vi "RT Initialize Input Image (SubVI).vi"(8 "error in (no error)":errorcluster, 10 "Image Type":T2 items=["Grayscale (U8)", "Grayscale (I16)", "Grayscale (SGL)", "Complex (CSG)", "RGB (U32)", "HSL (U32)", "RGB (U64)", "Grayscale (U16)"], 11 "Image Size In":T1) -> (0 "error out":errorcluster, 2 "Input Image Size Out":T1, 3 "Input Image Out":T3)   [LabVIEW 2017]
uses:
  Controls/Image Size.ctl
  <vilib>/vision/Image Controls.llb/IMAQ Image.ctl
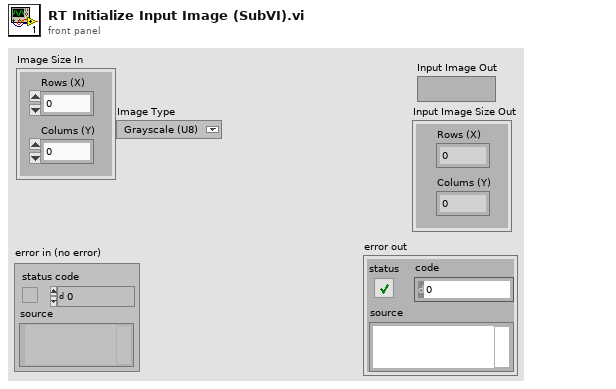
[diagram p1: front panel]
types:
  T1 = typedef "Image Size.ctl" = cluster{"Rows (X)":u16, "Colums (Y)":u16}
  T2 = typedef "Image Type" = u32
  T3 = typedef "IMAQ Image.ctl" = refnum<image>
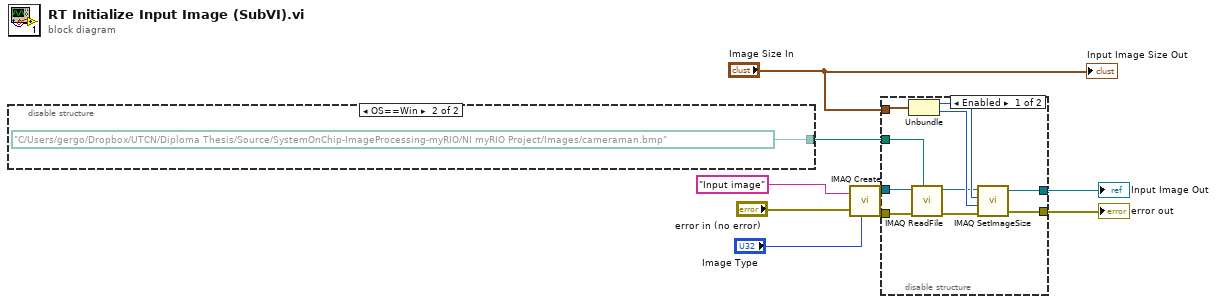
[diagram p0: block diagram]
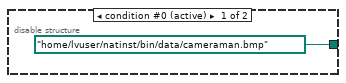
[diagram p2: hidden frame]
diagram:
  n1 = disable-structure shown="OS==Win" {
    disable-tunnel: [path "/home/lvuser/natinst/bin/data/cameraman.bmp" ("File Path") path "C:/Users/gergo/Dropbox/UTCN/Diploma Thesis/Source/SystemOnChip-ImageProcessing-myRIO/NI myRIO Project/Images/cameraman.bmp" ("File Path")] -> w1
    frame condition #0 (active) {
    }
    frame condition #1 {
    }
  }
  n2 = call "IMAQ Create"("Image Name"="Input image", "Image Type"="Image Type", "error in (no error)"="error in (no error)") -> ("New Image"=w4:T3, "error out"=w3:errorcluster)  [unwired: 2 in]
  n3 = disable-structure shown="Enabled" {
    disable-tunnel: "Image Size In" -> [w19 _]
    disable-tunnel: [w18 w23] -> w8
    disable-tunnel: [w16 w22] -> w7
    disable-tunnel: w4 -> [w14 w23]
    disable-tunnel: w3 -> [w13 w22]
    disable-tunnel: w1 -> [w12 _]
    frame Enabled {
      n4 = Unbundle(w19) -> ("Rows (X)"=w20:u16, "Colums (Y)"=w21:u16)
      n5 = call "IMAQ ReadFile"("File Path"=w12, "error in (no error)"=w13, "Image"=w14) -> ("error out"=w15:errorcluster, "Image Out"=w17:T3)  [unwired: 4 in, 3 out]
      n6 = call "IMAQ SetImageSize"("error in (no error)"=w15, "Y Resolution"=w21, "X Resolution"=w20, "Image"=w17) -> ("error out"=w16:errorcluster, "Image Out"=w18:T3)  [unwired: 1 in]
    }
    frame Disabled {
    }
  }
  "Input Image Out" <- w8
  "error out" <- w7
  "Input Image Size Out" <- "Image Size In"
